vi "01_simple_frequency_sweep.vi"() -> ()   [LabVIEW 2010]
uses:
  <vilib>/Instr/_visa.llb/VISA Open Access Mode.ctl
panel:
  out "Start Frequency":dbl format="%#_6p"
  out "Stop Frequency":dbl format="%#_6p"
  in  "Data Format D":string(combo)="LOGMAG"
  in  "Port Data D":string(combo)="S22,"
  in  "Data Format C":string(combo)="LOGMAG"
  in  "Port Data C":string(combo)="S12,"
  in  "Data Format B":string(combo)="LOGMAG"
  in  "Port Data B":string(combo)="S21,"
  in  "Data Format A":string(combo)="LOGMAG"
  in  "Port Data A":string(combo)="S11,"
  out "Plot B 2":cluster{"X":dbl[], "Y":dbl[]}[](graph)
  out "Plot A 2":cluster{"X":dbl[], "Y":dbl[]}[](graph)
  out "Plot B":cluster{"X":dbl[], "Y":dbl[]}[](graph)
  out "C return count":u32
  out "D return count":u32
  out "B return count":u32
  out "Plot A":cluster{"X":dbl[], "Y":dbl[]}[](graph)
  out "FORMAT read buffer":string="\nOK\n-9.1380180522471278e+01,-8.7561871955884968e+01,-9.3857206221490159e+01,-8.6858133994421038e+01,-9.2478674113988177e+01,-9.0923276531138669e+01,-8.5412713079243062e+01,-1.0680557752551536e+02,-9.8139396247310913e+01,-9.5942388317685925e+01,-8.8070150545760754e+01,-8.6010589064907776e+01,-8.1381403758226128e+01,-8.8612193914124816e+01,-8.8234033228500678e+01,-8.6784736973470515e+01,-8.8390475151936997e+01,-9.0166894093978101e+01,-9.3235516052204275e+01,-9.8498375048397122e+01,-8.9926362074673008e+01,-9.3883535338797174e+01,-9.4616326611874769e+01,-9.1184197705494796e+01,-8.2469727001096260e+01,-9.0246555044546454e+01,-8.5790709978521434e+01,-9.1210294324322035e+01,-9.1528412207460946e+01,-9.1774544150860308e+01,-8.6907110149069169e+01,-8.8657427293260227e+01,-8.3588468477941632e+01,-7.9449634296824570e+01,-8.4863492045148632e+01,-7.7255650086811954e+01,-8.0333893002109264e+01,-8.2062899737639611e+01,-8.9239718140047231e+01,-9.2058942343243828e+01,-8.7435414845914735e+01,-9.2380670007406280e+01,-8.6647335"
  out "INIT read buffer":string="\nOK\n-9.1380180522471278e+01,-8.7561871955884968e+01,-9.3857206221490159e+01,-8.6858133994421038e+01,-9.2478674113988177e+01,-9.0923276531138669e+01,-8.5412713079243062e+01,-1.0680557752551536e+02,-9.8139396247310913e+01,-9.5942388317685925e+01,-8.8070150545760754e+01,-8.6010589064907776e+01,-8.1381403758226128e+01,-8.8612193914124816e+01,-8.8234033228500678e+01,-8.6784736973470515e+01,-8.8390475151936997e+01,-9.0166894093978101e+01,-9.3235516052204275e+01,-9.8498375048397122e+01,-8.9926362074673008e+01,-9.3883535338797174e+01,-9.4616326611874769e+01,-9.1184197705494796e+01,-8.2469727001096260e+01,-9.0246555044546454e+01,-8.5790709978521434e+01,-9.1210294324322035e+01,-9.1528412207460946e+01,-9.1774544150860308e+01,-8.6907110149069169e+01,-8.8657427293260227e+01,-8.3588468477941632e+01,-7.9449634296824570e+01,-8.4863492045148632e+01,-7.7255650086811954e+01,-8.0333893002109264e+01,-8.2062899737639611e+01,-8.9239718140047231e+01,-9.2058942343243828e+01,-8.7435414845914735e+01,-9.2380670007406280e+01,-8.6647335"
  out "SWEep:POINts? read buffer":string
  out "A return count":u32
  out "IDN read buffer":string
  out "error out":errorcluster={"status"=FALSE, "code"=1073676294, "source"="VISA Read in VNA5 SCPI test_2024test1.vi"}
  in  "error in (no error)":errorcluster
  # "NOTE: VNA5 Software must be running for SCPI Interface (and connected to Demo or Real Device)"
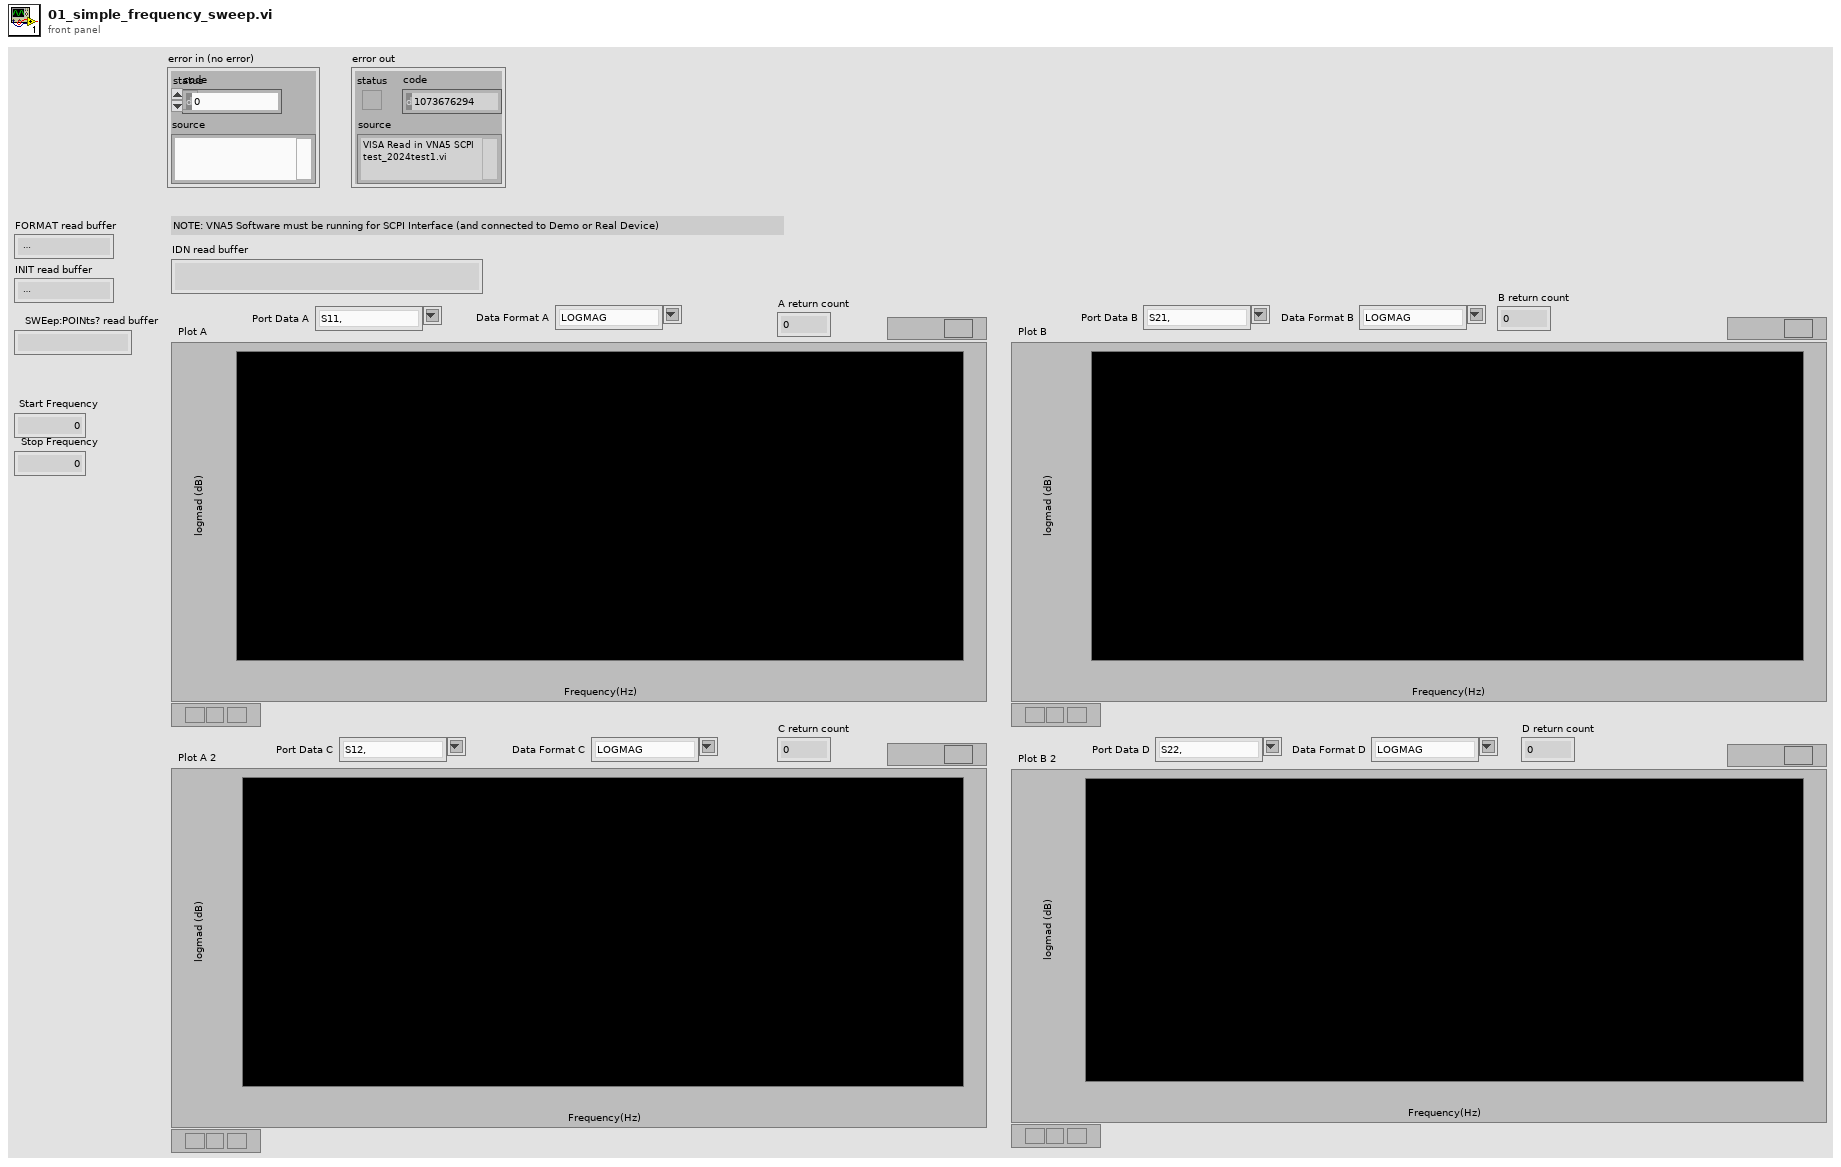
[diagram p1: front panel]
types:
  T1 = typedef "VISA Open Access Mode.ctl" = u32
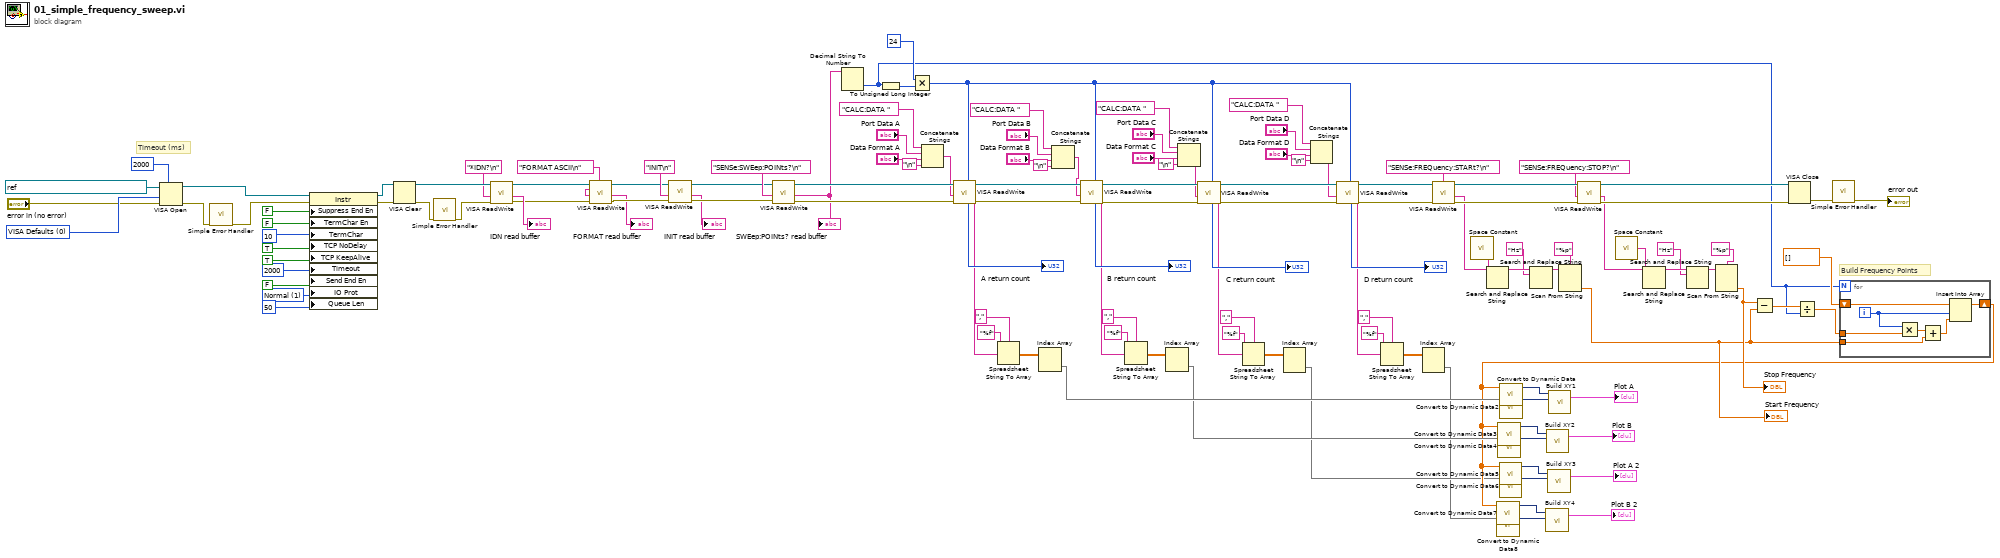
[diagram p0: block diagram]
diagram:
  w64 = u16 1 items=["Normal"=1, "VXI/FDC"=2, "GPIB/HS488"=3, "Serial-TCPIP-USB/488 Strings"=4, "USBTMC/Vendor-Specific"=5] ("Message Based Settings:IO Protocol")
  w127 = T1 0 items=["VISA Defaults"=0, "Exclusive Lock"=1, "Load Configured Settings"=4] ("Access Mode")
  # "Build Frequency Points"
  # "Timeout (ms)"
  n1 = VISA Open(timeout (0)=u32 2000 ("VISA Open timeout (0)"), access mode=w127, error in (no error)="error in (no error)", VISA resource name=refnum<visa-resource-name> "TCPIP0::127.0.0.1::5025::SOCKET") -> (VISA resource name=w128:refnum<visa-resource-name>, error out=w71:errorcluster)  [unwired: 1 in]
  n2 = call <vilib>:"Simple Error Handler.vi"("error in (no error)"=w71) -> ("error out"=w70:errorcluster)  [unwired: 4 in, 4 out]
  n3 = property class="Instr"(reference=w128, error in=w70, "Suppress End En"=FALSE, "TermChar En"=FALSE ("Message Based Settings:Termination Character Enable"), "TermChar"=u8 10 ("Message Based Settings:Termination Character"), "TCP NoDelay"=TRUE ("TCP/IP Settings:No Packet Delay"), "TCP KeepAlive"=TRUE ("TCP/IP Settings:Keep-Alive Packets"), "Timeout"=u32 2000 ("General Settings:Timeout Value"), "Send End En"=FALSE ("Message Based Settings:Send End Enable"), "IO Prot"=w64, "Queue Len"=u32 50 ("General Settings:Maximum Queue Length")) -> (reference out=w124:refnum<visa-resource-name>, error out=w123:errorcluster)
  n4 = VISA Clear(VISA resource name=w124, error in (no error)=w123) -> (VISA resource name out=w112:refnum<visa-resource-name>, error out=w60:errorcluster)
  n5 = call <vilib>:"Simple Error Handler.vi"("error in (no error)"=w60) -> ("error out"=w59:errorcluster)  [unwired: 4 in, 4 out]
  n6 = call "VISA ReadWrite.vi"("error in (no error)"=w59, "write buffer"="*IDN?\n", "VISA Refnum in"=w112) -> ("error out"=w107:errorcluster, "read buffer"=→"IDN read buffer":string, "VISA Refnum out"=w106:refnum<visa-resource-name>)  [unwired: 4 in, 2 out]
  n7 = call "VISA ReadWrite.vi"("error in (no error)"=w107, "write buffer"="FORMAT ASCII\n", "VISA Refnum in"=w106) -> ("error out"=w109:errorcluster, "read buffer"=→"FORMAT read buffer":string, "VISA Refnum out"=w108:refnum<visa-resource-name>)  [unwired: 4 in, 2 out]
  n8 = call "VISA ReadWrite.vi"("error in (no error)"=w109, "write buffer"="INIT\n", "VISA Refnum in"=w108) -> ("error out"=w118:errorcluster, "read buffer"=→"INIT read buffer":string, "VISA Refnum out"=w117:refnum<visa-resource-name>)  [unwired: 4 in, 2 out]
  n9 = call "VISA ReadWrite.vi"("error in (no error)"=w118, "write buffer"="SENSe:SWEep:POINts?\n", "VISA Refnum in"=w117) -> ("error out"=w120:errorcluster, "read buffer"=w115:string, "VISA Refnum out"=w121:refnum<visa-resource-name>)  [unwired: 4 in, 2 out]
  "SWEep:POINts? read buffer" <- w115
  n10 = Decimal String To Number(string=w115) -> (number=w72:i32)  [unwired: 2 in, 1 out]
  n11 = To Unsigned Long Integer(number=w72) -> (unsigned 32bit integer=w73:u32)
  n12 = Multiply(x=u32 24, y=w73) -> (x*y=w37:u32)
  n13 = Concatenate Strings("CALC:DATA " ("write buffer"), "Port Data A", "Data Format A", "\n") -> (w16:string)
  n14 = call "VISA ReadWrite.vi"("Read byte count"=w37, "error in (no error)"=w120, "write buffer"=w16, "VISA Refnum in"=w121) -> ("error out"=w52:errorcluster, "read buffer"=w100:string, "VISA Refnum out"=w53:refnum<visa-resource-name>, "Read return count"=→"A return count":u32)  [unwired: 3 in, 1 out]
  n15 = Spreadsheet String To Array(delimiter (Tab)=",", format string="%f", spreadsheet string=w100) -> (array=w101:dbl[][])  [unwired: 1 in]
  n16 = Index Array(array=w101) -> (element=w34:dbl[])  [unwired: 2 in]
  n17 = Concatenate Strings("CALC:DATA " ("write buffer"), "Port Data B", "Data Format B", "\n") -> (w3:string)
  n18 = call "VISA ReadWrite.vi"("Read byte count"=w37, "error in (no error)"=w52, "write buffer"=w3, "VISA Refnum in"=w53) -> ("error out"=w41:errorcluster, "read buffer"=w54:string, "VISA Refnum out"=w40:refnum<visa-resource-name>, "Read return count"=→"B return count":u32)  [unwired: 3 in, 1 out]
  n19 = Spreadsheet String To Array(delimiter (Tab)=",", format string="%f", spreadsheet string=w54) -> (array=w55:dbl[][])  [unwired: 1 in]
  n20 = Index Array(array=w55) -> (element=w30:dbl[])  [unwired: 2 in]
  n21 = Concatenate Strings("CALC:DATA " ("write buffer"), "Port Data C", "Data Format C", "\n") -> (w2:string)
  n22 = call "VISA ReadWrite.vi"("Read byte count"=w37, "error in (no error)"=w41, "write buffer"=w2, "VISA Refnum in"=w40) -> ("error out"=w38:errorcluster, "read buffer"=w42:string, "VISA Refnum out"=w39:refnum<visa-resource-name>, "Read return count"=→"C return count":u32)  [unwired: 3 in, 1 out]
  n23 = Spreadsheet String To Array(delimiter (Tab)=",", format string="%f", spreadsheet string=w42) -> (array=w43:dbl[][])  [unwired: 1 in]
  n24 = Index Array(array=w43) -> (element=w22:dbl[])  [unwired: 2 in]
  n25 = Concatenate Strings("CALC:DATA " ("write buffer"), "Port Data D", "Data Format D", "\n") -> (w1:string)
  n26 = call "VISA ReadWrite.vi"("Read byte count"=w37, "error in (no error)"=w38, "write buffer"=w1, "VISA Refnum in"=w39) -> ("error out"=w35:errorcluster, "read buffer"=w47:string, "VISA Refnum out"=w36:refnum<visa-resource-name>, "Read return count"=→"D return count":u32)  [unwired: 3 in, 1 out]
  n27 = Spreadsheet String To Array(delimiter (Tab)=",", format string="%f", spreadsheet string=w47) -> (array=w48:dbl[][])  [unwired: 1 in]
  n28 = Index Array(array=w48) -> (element=w21:dbl[])  [unwired: 2 in]
  n29 = call "VISA ReadWrite.vi"("error in (no error)"=w35, "write buffer"="SENSe:FREQuency:STARt?\n", "VISA Refnum in"=w36) -> ("error out"=w99:errorcluster, "read buffer"=w89:string, "VISA Refnum out"=w96:refnum<visa-resource-name>)  [unwired: 4 in, 2 out]
  n30 = call <vilib>:"Space Constant.vi"() -> ("String"=w88:string)
  n31 = Search and Replace String(input string=w89, search string=w88) -> (result string=w87:string)  [unwired: 6 in, 3 out]
  n32 = call "Convert to Dynamic Data8"("Array"=w21) -> ("Dynamic Data Type"=w24:dynamicdata)  [unwired: 3 in]
  n33 = call "Convert to Dynamic Data4"("Array"=w30) -> ("Dynamic Data Type"=w31:dynamicdata)  [unwired: 3 in]
  n34 = call "Convert to Dynamic Data6"("Array"=w22) -> ("Dynamic Data Type"=w27:dynamicdata)  [unwired: 3 in]
  n35 = call "Convert to Dynamic Data2"("Array"=w34) -> ("Dynamic Data Type"=w91:dynamicdata)  [unwired: 3 in]
  n36 = Search and Replace String(input string=w87, search string="Hz") -> (result string=w85:string)  [unwired: 6 in, 3 out]
  n37 = Scan From String(format string="%p" ("input string"), input string=w85) -> (output 1=w74:dbl)  [unwired: 3 in, 3 out]
  "Start Frequency" <- w74
  n38 = call "VISA ReadWrite.vi"("error in (no error)"=w99, "write buffer"="SENSe:FREQuency:STOP?\n", "VISA Refnum in"=w96) -> ("error out"=w98:errorcluster, "read buffer"=w80:string, "VISA Refnum out"=w97:refnum<visa-resource-name>)  [unwired: 4 in, 2 out]
  n39 = call <vilib>:"Space Constant.vi"() -> ("String"=w84:string)
  n40 = Search and Replace String(input string=w80, search string=w84) -> (result string=w83:string)  [unwired: 6 in, 3 out]
  n41 = Search and Replace String(input string=w83, search string="Hz") -> (result string=w81:string)  [unwired: 6 in, 3 out]
  n42 = Scan From String(format string="%p" ("input string"), input string=w81) -> (output 1=w75:dbl)  [unwired: 3 in, 3 out]
  "Stop Frequency" <- w75
  n43 = Subtract(x=w75, y=w74) -> (x-y=w77:dbl)
  n44 = VISA Close(VISA resource name=w97, error in (no error)=w98) -> (error out=w130:errorcluster)
  n45 = Divide(x=w77, y=w72) -> (x/y=w76:dbl)
  n46 = call <vilib>:"Simple Error Handler.vi"("error in (no error)"=w130) -> ("error out"=→"error out":errorcluster)  [unwired: 4 in, 4 out]
  n47 = for {
    N: w72 -> [_]
    shift-right: [w138] -> w23
    shift-left: dbl[] [] ("array") -> [w137]
    tunnel: w76 -> [w135]
    tunnel: w74 -> [w136]
    i -> [w132]
    n48 = Multiply(x=w132, y=w135) -> (x*y=w133:dbl)
    n49 = Add(x=w133, y=w136) -> (x+y=w134:dbl)
    n50 = Insert Into Array(array=w137, index=w132, new element=w134) -> (w138:dbl[])
  }
  n51 = call "Convert to Dynamic Data7"("Array"=w23) -> ("Dynamic Data Type"=w25:dynamicdata)  [unwired: 3 in]
  n52 = call "Convert to Dynamic Data3"("Array"=w23) -> ("Dynamic Data Type"=w32:dynamicdata)  [unwired: 3 in]
  n53 = call "Convert to Dynamic Data5"("Array"=w23) -> ("Dynamic Data Type"=w28:dynamicdata)  [unwired: 3 in]
  n54 = call "Convert to Dynamic Data"("Array"=w23) -> ("Dynamic Data Type"=w92:dynamicdata)  [unwired: 3 in]
  n55 = call "Build XY4"("Y Input"=w24, "X Input"=w25) -> ("XY Graph"=→"Plot B 2":cluster{"X":dbl[], "Y":dbl[]}[])  [unwired: 8 in, 1 out]
  n56 = call "Build XY2"("Y Input"=w31, "X Input"=w32) -> ("XY Graph"=→"Plot B":cluster{"X":dbl[], "Y":dbl[]}[])  [unwired: 8 in, 1 out]
  n57 = call "Build XY3"("Y Input"=w27, "X Input"=w28) -> ("XY Graph"=→"Plot A 2":cluster{"X":dbl[], "Y":dbl[]}[])  [unwired: 8 in, 1 out]
  n58 = call "Build XY1"("Y Input"=w91, "X Input"=w92) -> ("XY Graph"=→"Plot A":cluster{"X":dbl[], "Y":dbl[]}[])  [unwired: 8 in, 1 out]
